vi "Initialisation commands from excel file.vi"(11 "Filepath Program code":path[](array[path])=[path "C:/Users/aguillaume3/Desktop/LabVIEW for Chemical Profiles in Liquid Exchanger/20190530_SequenceChemicalProfile_Liquid_Exchanger.xlsx"]) -> (1 "Step list":string[](array[string]), 2 "Fragmentation commands for waiting times":cluster{"subarray 2":dbl[]}[](array[cluster]), 3 "Fragmentation commands for pressure":cluster{"subarray 2":dbl[][]}[](array[cluster]))   [LabVIEW 2019]
panel:
  out "index init":i32
  out "index end":i32
  out "String":string
  out "Step Label":string[](array[string])
  out "Size step label":i32
  out "Size Command Waiting Times":i32
  out "Size Command Pressures":i32[](array[numeric])
  out "Command Waiting Times (s)":dbl[](array[numeric])
  out "Command Pressures":dbl[][](array[numeric])
  # "Inputs"
  # "Outputs"
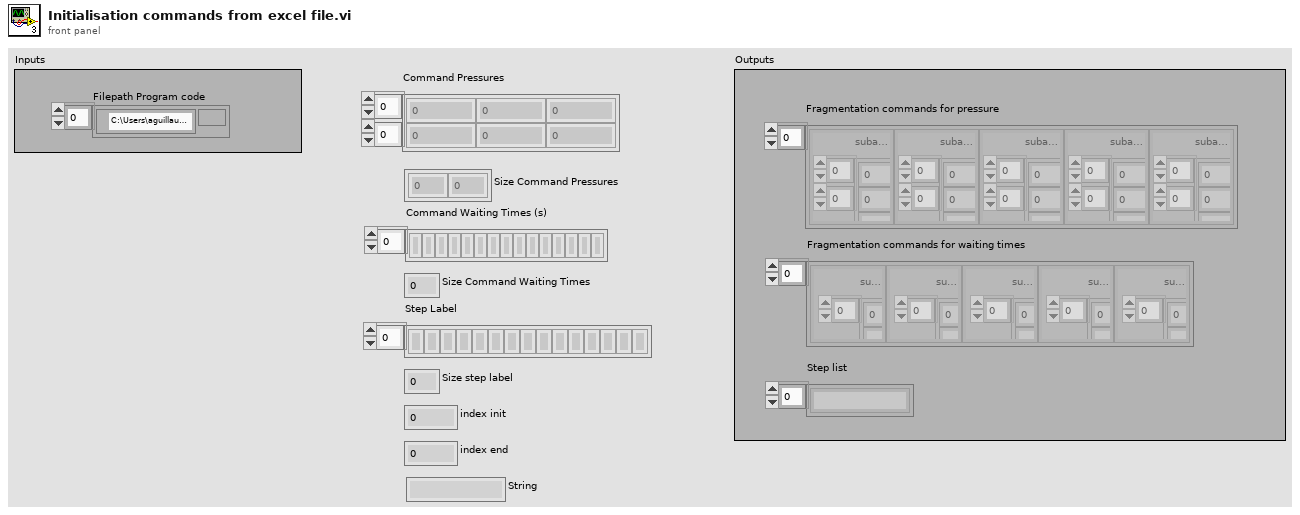
[diagram p1: front panel]
types:
  T1 = cluster{"Start row":i32, "Start col":i32, "End row":i32, "End col":i32}
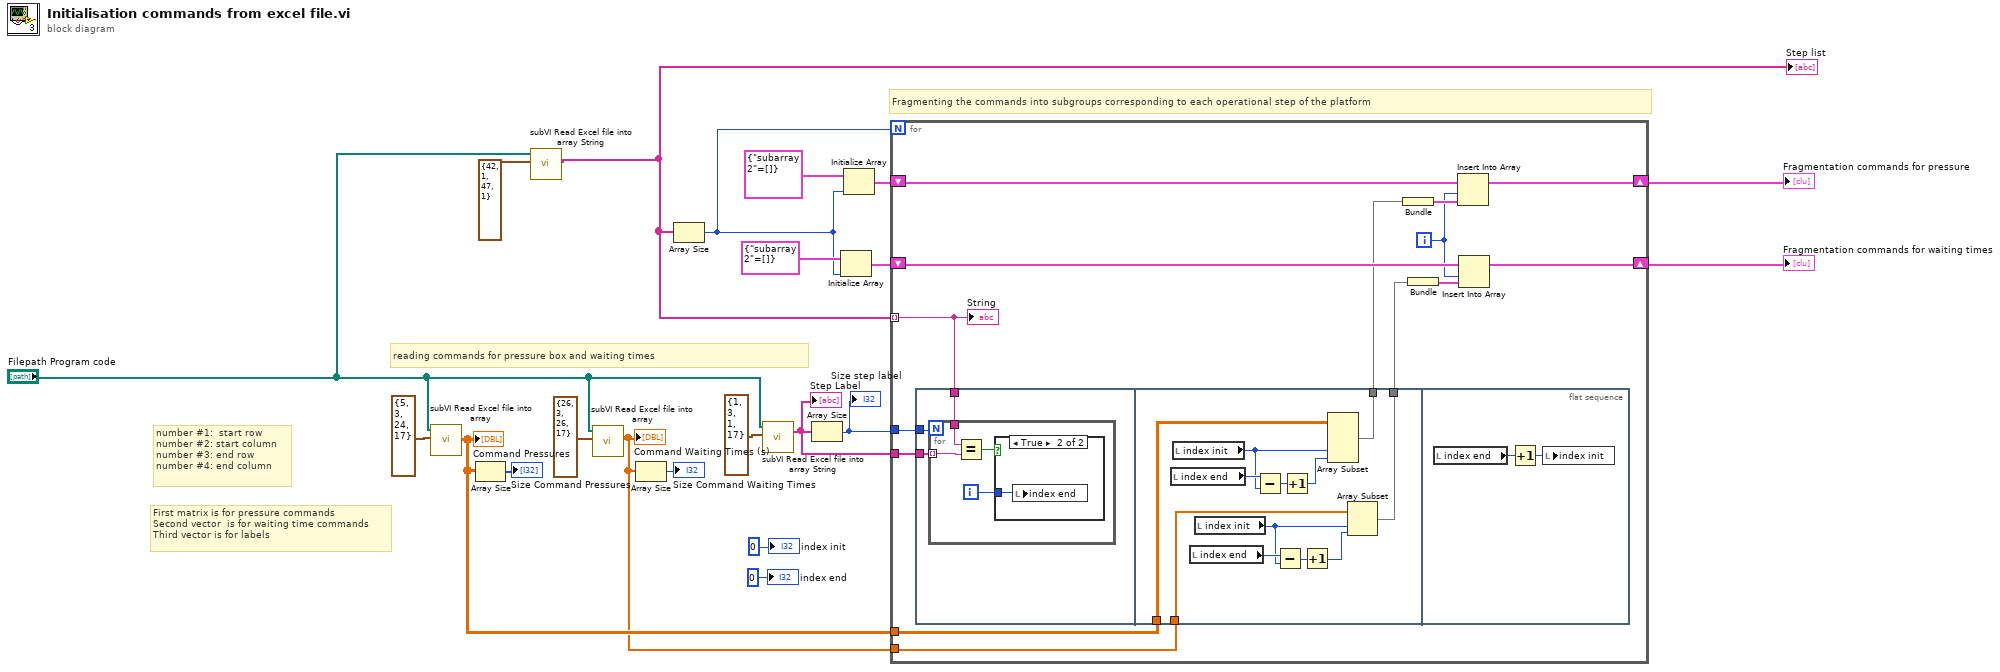
[diagram p0: block diagram]
diagram:
  # "First matrix is for pressure commands\nSecond vector  is for waiting time commands\nThird vector is for labels"
  # "number #1:  start row\nnumber #2: start column \nnumber #3: end row\nnumber #4: end column"
  # "Fragmenting the commands into subgroups corresponding to each operational step of the platform"
  # "reading commands for pressure box and waiting times"
  n1 = call "subVI Read Excel file into array.vi"("Select row & col to read"=T1 {"Start row"=5, "Start col"=3, "End row"=24, "End col"=17}, "Filepath"="Filepath Program code") -> ("2D matrix output"=w14:dbl[][])  [unwired: 8 in, 1 out]
  "Command Pressures" <- w14
  n2 = Array Size(array=w14) -> (size(s)=→"Size Command Pressures":i32[])
  n3 = call "subVI Read Excel file into array String.vi"("Select row & col to read"=T1 {"Start row"=42, "Start col"=1, "End row"=47, "End col"=1}, "Filepath"="Filepath Program code") -> ("array 2"=w2:string[])  [unwired: 8 in, 1 out]
  "Step list" <- w2
  n4 = call "subVI Read Excel file into array.vi"("Select row & col to read"=T1 {"Start row"=26, "Start col"=3, "End row"=26, "End col"=17}, "Filepath"="Filepath Program code") -> ("1D vector output"=w8:dbl[])  [unwired: 8 in, 1 out]
  "Command Waiting Times (s)" <- w8
  n5 = Array Size(array=w8) -> (size(s)=→"Size Command Waiting Times":i32)
  n6 = Array Size(array=w2) -> (size(s)=w5:i32)
  n7 = call "subVI Read Excel file into array String.vi"("Select row & col to read"=T1 {"Start row"=1, "Start col"=3, "End row"=1, "End col"=17}, "Filepath"="Filepath Program code") -> ("array 2"=w15:string[])  [unwired: 8 in, 1 out]
  "Step Label" <- w15
  n8 = Array Size(array=w15) -> (size(s)=w16:i32)
  "Size step label" <- w16
  n9 = Initialize Array(cluster{"subarray 2":dbl[]} {"subarray 2"=[]}, w5) -> (w7:cluster{"subarray 2":dbl[]}[])
  n10 = Initialize Array(cluster{"subarray 2":dbl[][]} {"subarray 2"=[]}, w5) -> (w11:cluster{"subarray 2":dbl[][]}[])
  n11 = for {
    N: w5 -> [_]
    tunnel: w2 -> [w33] mode=indexing
    tunnel: w16 -> [w35]
    tunnel: w15 -> [w34]
    tunnel: w14 -> [w32]
    shift-right: [w31] -> w10
    shift-left: w11 -> [w30]
    tunnel: w8 -> [w29]
    shift-right: [w28] -> w6
    shift-left: w7 -> [w27]
    i -> [w22]
    n12 = flat-sequence {
      tunnel: w35 -> [w38]
      tunnel: w34 -> [w37]
      tunnel: w33 -> [w36]
      tunnel: w32 -> [w55]
      tunnel: [w50] -> w24
      tunnel: w29 -> [w47]
      tunnel: [w44] -> w23
      frame #0 {
        n13 = for {
          N: w38 -> [_]
          tunnel: w37 -> [w42] mode=indexing
          tunnel: w36 -> [w41]
          i -> [w39]
          n14 = Equal?(x=w41, y=w42) -> (x = y?=w40:bool)
          n15 = case shown="True" w40 {
            tunnel: w39 -> [_ w43]
            frame False {
            }
            frame True {
              n16 = local write "index end"(w43) -> ()
            }
          }
        }
      }
      frame #1 {
        n17 = local read "index end"() -> (w54:i32)
        n18 = local read "index init"() -> (w53:i32)
        n19 = local read "index end"() -> (w48:i32)
        n20 = local read "index init"() -> (w45:i32)
        n21 = Subtract(x=w54, y=w53) -> (x-y=w52:i32)
        n22 = Subtract(x=w48, y=w45) -> (x-y=w49:i32)
        n23 = Increment(x=w52) -> (x+1=w51:i32)
        n24 = Increment(x=w49) -> (x+1=w46:i32)
        n25 = Array Subset(array=w55, index (col)=w53, length (col)=w51) -> (w50:dbl[][])  [unwired: 2 in]
        n26 = Array Subset(array=w47, index=w45, length=w46) -> (w44:dbl[])
      }
      frame #2 {
        n27 = local read "index end"() -> (w56:i32)
        n28 = Increment(x=w56) -> (x+1=w57:i32)
        n29 = local write "index init"(w57) -> ()
      }
    }
    n30 = Bundle(w24) -> (w26:cluster{dbl[][]})  [unwired: 1 in]
    n31 = Bundle(w23) -> (w25:cluster{dbl[]})  [unwired: 1 in]
    n32 = Insert Into Array(array=w30, index=w22, new element=w26) -> (w31:cluster{"subarray 2":dbl[][]}[])
    n33 = Insert Into Array(array=w27, index=w22, new element=w25) -> (w28:cluster{"subarray 2":dbl[]}[])
    "String" <- w33
  }
  "Fragmentation commands for pressure" <- w10
  "Fragmentation commands for waiting times" <- w6
  "index init" <- 0 ("index")
  "index end" <- 0 ("counter")
